vi "Dual DM Control - MAIN V2.vi"() -> ()   [LabVIEW 2014]
uses:
  DMControl_V3.ctl
  <vilib>/Utility/file.llb/Write To Spreadsheet File (DBL).vi
panel:
  in  "Top Mirror":T1 {"Modes"."Amplititude" step=0.05}
  in  "Bottom Mirror":T1 {"Modes"."Amplititude" step=0.05}
  in  "Stop":bool
  out "Top Mirror":dbl[][](graph)
  out "Bottom Mirror":dbl[][](graph)
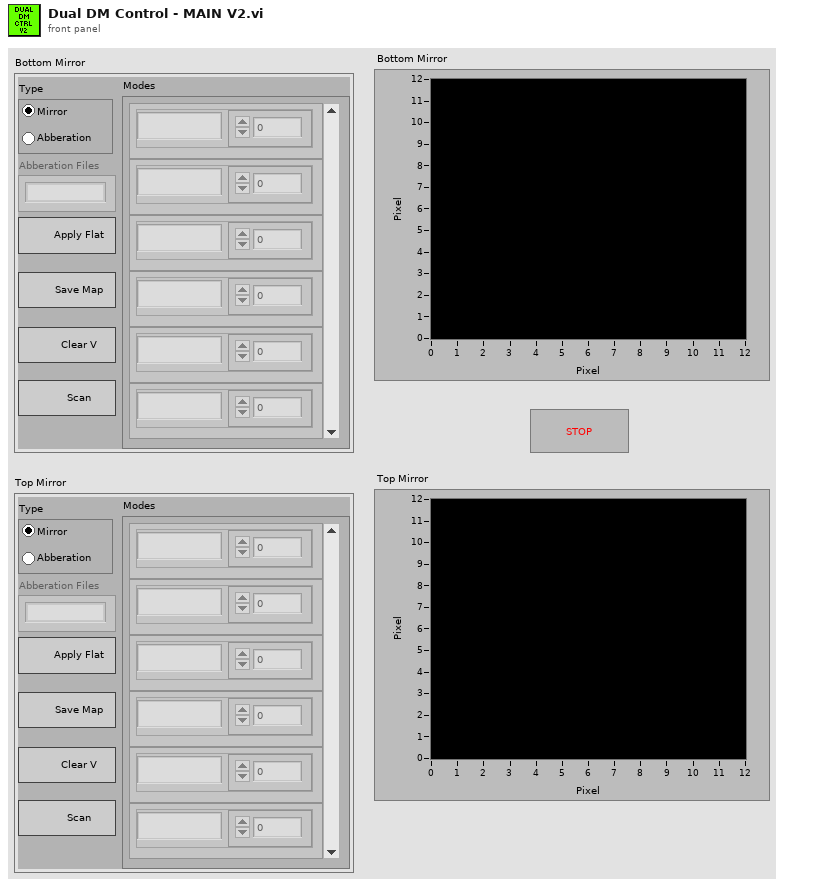
[diagram p1: front panel]
types:
  T1 = typedef "DMControl_V3.ctl" = cluster{"Type":enum32{"Mirror", "Abberation"}, "Modes":cluster{"Mode":string, "Amplititude":dbl}[], "Apply Flat":bool, "Save Map":bool, "Clear Voltage":bool, "Abberation Files":u16, "Scan ":bool}
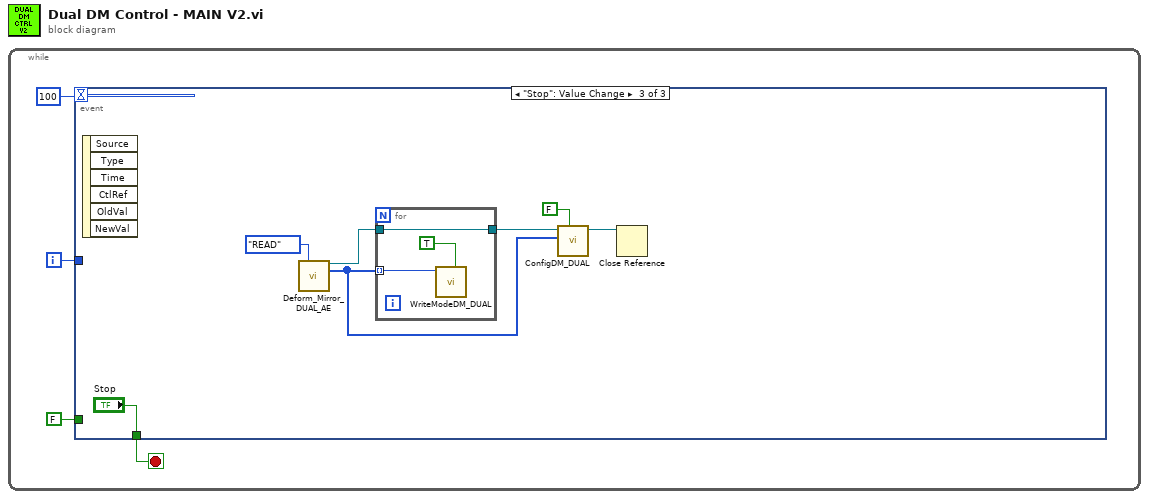
[diagram p0: block diagram]
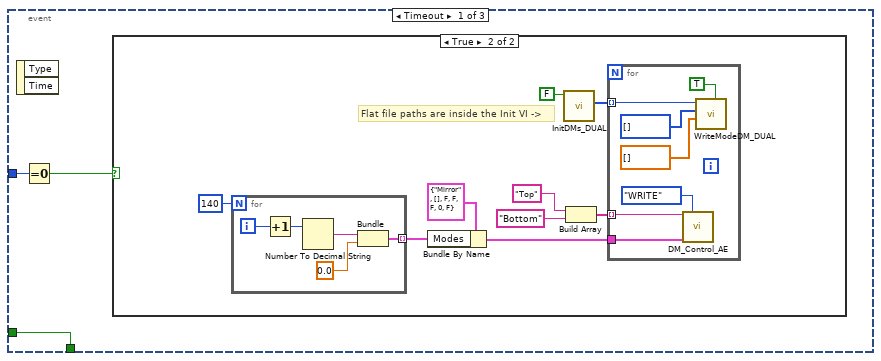
[diagram p2: hidden frame]
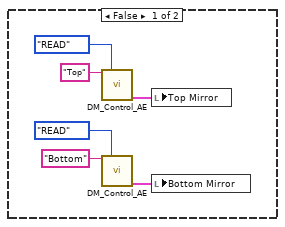
[diagram p3: hidden frame]
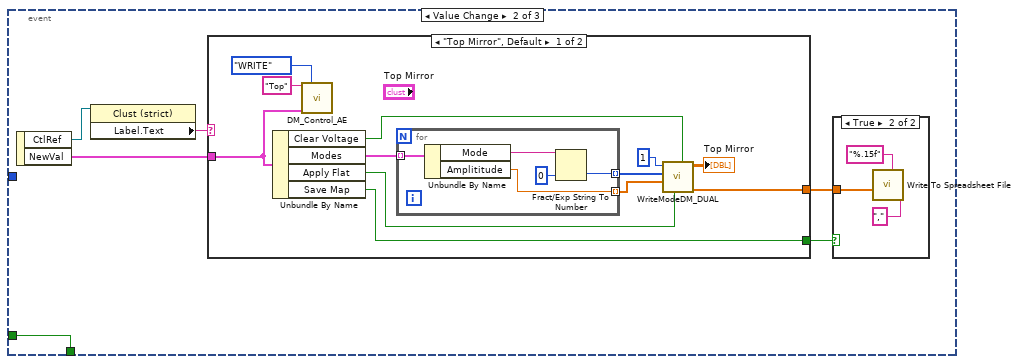
[diagram p4: hidden frame]
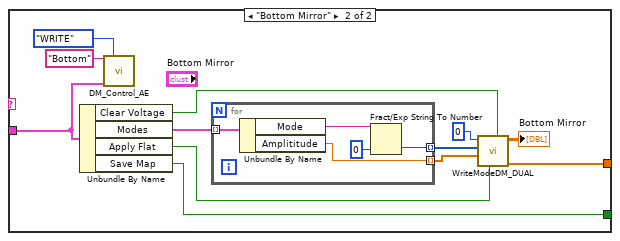
[diagram p6: hidden frame]
diagram:
  n1 = while {
    i -> [w1]
    stop <- w3 stop-if-true
    n2 = event shown="[2] \"Stop\": Value Change" {
      selector: _ -> [_ _ _]
      dyn-events: _ -> [_ _ _]
      timeout: 100 -> [_ _ _]
      tunnel: [w5 w40 "Stop"] -> w3
      tunnel: FALSE -> [w5 w40 _]
      tunnel: w1 -> [w7 _ _]
      event Timeout {
        n3 = event-data() -> ()  [unwired: 1 in, 2 out]
        n4 = Equal To 0?(x=w7) -> (x = 0?=w6:bool)
        n5 = case shown="True" w6 {
          frame False {
            n6 = call "DM_Control_AE.vi"("Mirror ID"="Top", "Action"=enum16{"WRITE", "READ"}."READ") -> ("Mirror Control OUT"=w9:T1)  [unwired: 12 in, 1 out]
            n7 = call "DM_Control_AE.vi"("Mirror ID"="Bottom", "Action"=enum16{"WRITE", "READ"}."READ") -> ("Mirror Control OUT"=w8:T1)  [unwired: 12 in, 1 out]
            n8 = local write "Top Mirror"(w9) -> ()
            n9 = local write "Bottom Mirror"(w8) -> ()
          }
          frame True {
            # "Flat file paths are inside the Init VI ->"
            n10 = for {
              N: 140 -> [_]
              tunnel: [w23] -> w21 mode=indexing
              i -> [w27]
              n11 = Increment(x=w27) -> (x+1=w26:i32)
              n12 = Number To Decimal String(number=w26) -> (decimal integer string=w25:string)  [unwired: 1 in]
              n13 = Bundle(w25, 0.0) -> (w23:cluster{string, dbl})  [unwired: 1 in]
            }
            n14 = Bundle By Name(cluster=T1 {"Type"=enum."Mirror", "Modes"=[], "Apply Flat"=FALSE, "Save Map"=FALSE, "Clear Voltage"=FALSE, "Abberation Files"=0, "Scan "=FALSE} ("Bottom Mirror"), "Modes"=w21) -> (w22:T1)
            n15 = call "InitDMs_DUAL.vi"("BM Flats"=FALSE) -> ("IDs"=w18:i32[])  [unwired: 9 in, 1 out]
            n16 = Build Array("Top" ("Mirror ID"), "Bottom" ("Mirror ID")) -> (w16:string[])
            n17 = for {
              tunnel: w18 -> [w34] mode=indexing
              tunnel: w16 -> [w29] mode=indexing
              tunnel: w22 -> [w28]
              n18 = call "DM_Control_AE.vi"("Mirror ID"=w29, "Action"=enum16{"WRITE", "READ"}."WRITE", "Mirror Control IN"=w28) -> ()  [unwired: 11 in, 2 out]
              n19 = call "WriteModeDM_DUAL.vi"("Clear DM Voltage"=TRUE, "Amplitudes"=dbl[] [], "Modes"=i32[] [], "Device"=w34) -> ()  [unwired: 6 in, 2 out]
            }
          }
        }
      }
      event Value Change {
        n20 = event-data() -> ("CtlRef"=w38:refnum<vi>, "NewVal"=w39:T1)  [unwired: 1 in]
        n21 = property class="Clust (strict)"(reference=w38) -> ("Label.Text"=w37:string)  [unwired: 1 in, 2 out]
        n22 = case shown="\"Top Mirror\", Default" w37 {
          tunnel: w39 -> [w46 w63]
          tunnel: [w45 w62] -> w36
          tunnel: [w44 w61] -> w35
          frame "Top Mirror", Default {
            n23 = Unbundle By Name(w46) -> ("Clear Voltage"=w51:bool, "Modes"=w54:cluster{"Mode":string, "Amplititude":dbl}[], "Apply Flat"=w50:bool, "Save Map"=w45:bool)
            n24 = call "DM_Control_AE.vi"("Mirror ID"="Top", "Action"=enum16{"WRITE", "READ"}."WRITE", "Mirror Control IN"=w46) -> ()  [unwired: 11 in, 2 out]
            n25 = for {
              tunnel: w54 -> [w60] mode=indexing
              tunnel: [w57] -> w53 mode=indexing
              tunnel: [w56] -> w52 mode=indexing
              n26 = Unbundle By Name(w60) -> ("Mode"=w58:string, "Amplititude"=w56:dbl)
              n27 = Fract/Exp String To Number(string=w58, default (0 dbl)=0) -> (number=w57:i32)  [unwired: 2 in, 1 out]
            }
            n28 = call "WriteModeDM_DUAL.vi"("Clear DM Voltage"=w51, "Flat File ON"=w50, "Amplitudes"=w52, "Modes"=w53, "Device"=1) -> ("Voltage Map Out"=w44:dbl[], "Voltage Map"=→"Top Mirror":dbl[][])  [unwired: 5 in]
          }
          frame "Bottom Mirror" {
            n29 = Unbundle By Name(w63) -> ("Clear Voltage"=w68:bool, "Modes"=w71:cluster{"Mode":string, "Amplititude":dbl}[], "Apply Flat"=w67:bool, "Save Map"=w62:bool)
            n30 = call "DM_Control_AE.vi"("Mirror ID"="Bottom", "Action"=enum16{"WRITE", "READ"}."WRITE", "Mirror Control IN"=w63) -> ()  [unwired: 11 in, 2 out]
            n31 = for {
              tunnel: w71 -> [w77] mode=indexing
              tunnel: [w74] -> w70 mode=indexing
              tunnel: [w73] -> w69 mode=indexing
              n32 = Unbundle By Name(w77) -> ("Mode"=w75:string, "Amplititude"=w73:dbl)
              n33 = Fract/Exp String To Number(string=w75, default (0 dbl)=0) -> (number=w74:i32)  [unwired: 2 in, 1 out]
            }
            n34 = call "WriteModeDM_DUAL.vi"("Clear DM Voltage"=w68, "Flat File ON"=w67, "Amplitudes"=w69, "Modes"=w70, "Device"=0) -> ("Voltage Map Out"=w61:dbl[], "Voltage Map"=→"Bottom Mirror":dbl[][])  [unwired: 5 in]
          }
        }
        n35 = case shown="True" w36 {
          tunnel: w35 -> [_ w41]
          frame False {
          }
          frame True {
            n36 = call-poly <vilib>:"Write To Spreadsheet File.vi"("delimiter (\\t)"="," ("delimiter (\\t)"), "format (%.3f)"="%.15f", "1D data"=w41) -> ()  [unwired: 5 in, 1 out]
          }
        }
      }
      event "Stop": Value Change {
        n37 = event-data() -> ()  [unwired: 1 in, 6 out]
        n38 = call "Deform_Mirror_DUAL_AE.vi"("Action"=enum16{"WRITE", "READ"}."READ") -> ("Refnum Out"=w82:refnum<k7>, "IDs Out"=w79:i32[])  [unwired: 10 in, 3 out]
        n39 = for {
          tunnel: w79 -> [w87] mode=indexing
          tunnel: w82 -> [w85]
          tunnel: [w85] -> w80
          n40 = call "WriteModeDM_DUAL.vi"("Clear DM Voltage"=TRUE, "Device"=w87) -> ()  [unwired: 8 in, 2 out]
        }
        n41 = call "ConfigDM_DUAL.vi"("High Voltage"=FALSE, "Dev IDs"=w79, "Automation Refnum in"=w80) -> ("Automation Refnum out"=w78:refnum<k7>)  [unwired: 7 in, 1 out]
        n42 = Close Reference(reference=w78) -> ()  [unwired: 1 in, 1 out]
      }
    }
  }
